vi "Get Max Range.vi"(8 "error in (no error)":errorcluster, 10 "Max Range In":T1, 11 "Plot Representation In":T2) -> (0 "error out":errorcluster, 2 "Max Range Out":T1, 3 "Plot Representation Out":T2)   [LabVIEW 2020, in "2D Plot Datatype.lvclass"]
uses:
  <vilib>/Math Plots/2D Math Plots/2D Plot/2D Plot Datatype/2D Plot Datatype.lvclass
  <vilib>/Math Plots/2D Math Plots/2D Plot/2D Plot/Typedef/Plot Representation.ctl
  <vilib>/Math Plots/2D Math Plots/2D Plot/2D Plot/Typedef/Range Cluster.ctl
  <vilib>/Math Plots/2D Math Plots/2D Plot/2D Plot/2D Plot.lvclass
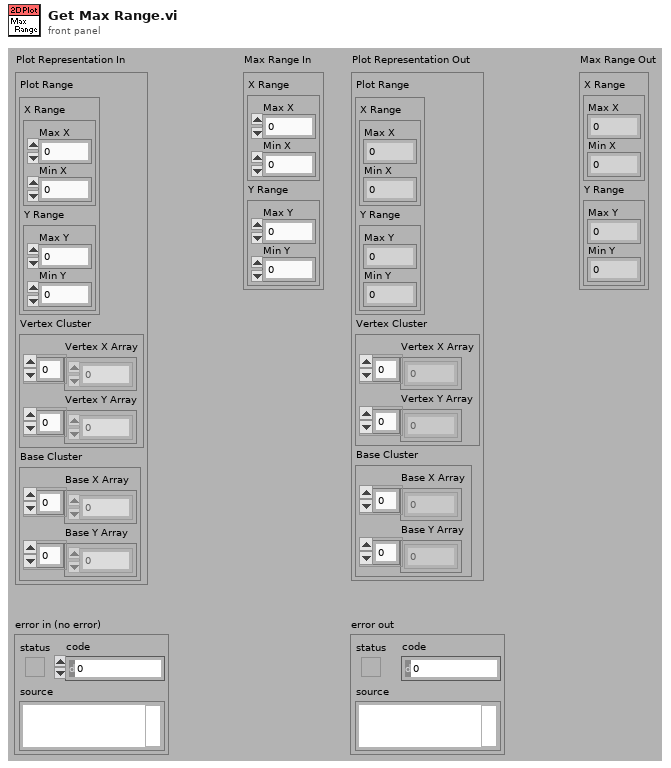
[diagram p1: front panel]
types:
  T1 = typedef "2D Plot.lvclass/Range Cluster.ctl" = cluster{"X Range":cluster{"Max X":dbl, "Min X":dbl}, "Y Range":cluster{"Max Y":dbl, "Min Y":dbl}}
  T2 = typedef "2D Plot.lvclass/Plot Representation.ctl" = cluster{"Plot Range":T1, "Vertex Cluster":cluster{"Vertex X Array":dbl[], "Vertex Y Array":dbl[]}, "Base Cluster":cluster{"Base X Array":dbl[], "Base Y Array":dbl[]}}
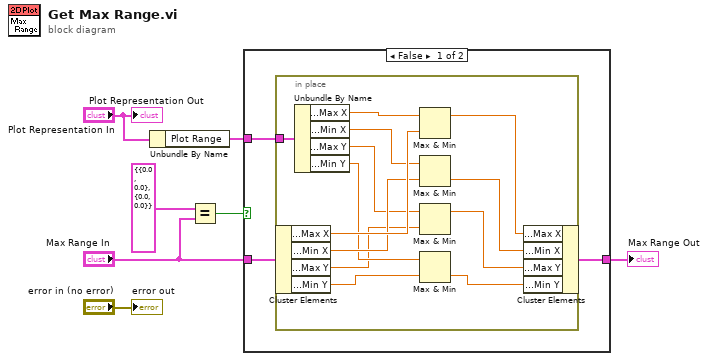
[diagram p0: block diagram]
diagram:
  n1 = Unbundle By Name("Plot Representation In") -> ("Plot Range"=w5:T1)
  n2 = Equal?(x=T1 {"X Range"={"Max X"=0.0, "Min X"=0.0}, "Y Range"={"Max Y"=0.0, "Min Y"=0.0}} ("Max Range In 2"), y="Max Range In") -> (x = y?=w7:bool)
  n3 = case shown="False" w7 {
    tunnel: "Max Range In" -> [w10 _]
    tunnel: w5 -> [w9 w24]
    tunnel: [w8 w24] -> w3
    frame False {
      n4 = in-place {
        in-place-border: w9 -> [w11]
        n5 = in-place-cluster #1(w10) -> ("X Range.Max X"=w22:dbl, "X Range.Min X"=w19:dbl, "Y Range.Max Y"=w13:dbl, "Y Range.Min Y"=w12:dbl)
        n6 = Unbundle By Name(w11) -> ("X Range.Max X"=w23:dbl, "X Range.Min X"=w20:dbl, "Y Range.Max Y"=w14:dbl, "Y Range.Min Y"=w15:dbl)
        n7 = Max & Min(x=w23, y=w22) -> (max(x,y)=w21:dbl)  [unwired: 1 out]
        n8 = Max & Min(x=w20, y=w19) -> (min(x,y)=w18:dbl)  [unwired: 1 out]
        n9 = Max & Min(x=w14, y=w13) -> (max(x,y)=w17:dbl)  [unwired: 1 out]
        n10 = Max & Min(x=w15, y=w12) -> (min(x,y)=w16:dbl)  [unwired: 1 out]
        n11 = in-place-cluster #1("X Range.Max X"=w21, "X Range.Min X"=w18, "Y Range.Max Y"=w17, "Y Range.Min Y"=w16) -> (w8:T1)
      }
    }
    frame True {
    }
  }
  "Max Range Out" <- w3
  "error out" <- "error in (no error)"
  "Plot Representation Out" <- "Plot Representation In"
